vi "Get Biometry Data Path.vi"(8 "error in (no error)":errorcluster caption="错误输入（无错误）", 9 "Display Parameter":T1(ring), 10 "condition":string, 11 "connection reference":T2) -> (0 "error out":errorcluster caption="错误输出", 2 "Data Path Output":string[](array[string]))   [LabVIEW 2015, in "Utility VIs.lvlib"]
doc: "该模板用于创建子VI。"
uses:
  Utility VIs.lvlib
  <vilib>/addons/database/Connection.llb/Conn ObjectReference.ctl
  Database Processing/Database Processing.lvlib
  <vilib>/addons/database/NI_Database_API.lvlib
panel:
  # "Busy"
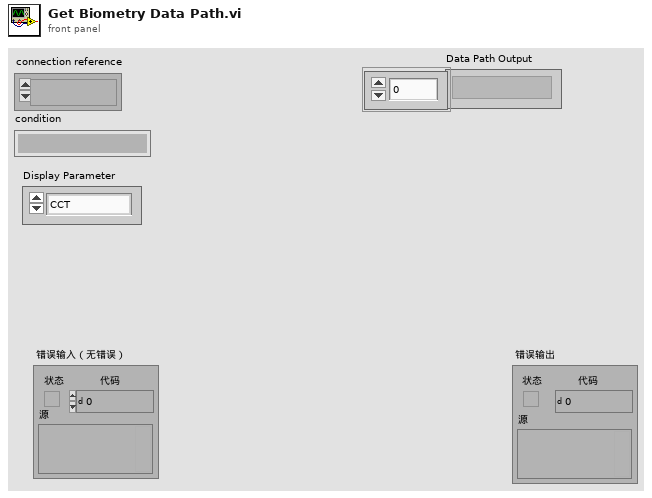
[diagram p1: front panel]
types:
  T1 = enum16{"CCT", "ACD", "LT", "RT", "AL", "PD", "WTW", "K_flat", "K_steep"}
  T2 = typedef "NI_Database_API.lvlib/Conn ObjectReference.ctl" = refnum<k1>
  T3 = typedef "Database Processing.lvlib/Biometry Attribute.ctl" = cluster{"Measure_ID":i64, "Measure_No":i64, "Ordinal":i64, "L_Or_R":string}
  T4 = typedef "Database Processing.lvlib/Biometry Data Path.ctl" = cluster{"Measure_ID":i64, "Ascan_data_Original":string, "picture_pupil_Original":string, "picture_WTW_Original":string, "Ascan_data_Processing":string, "picture_pupil_Processing":string, "picture_WTW_Processing":string, "picture_Processing_K":string, "picture_Processing_ALL":string}
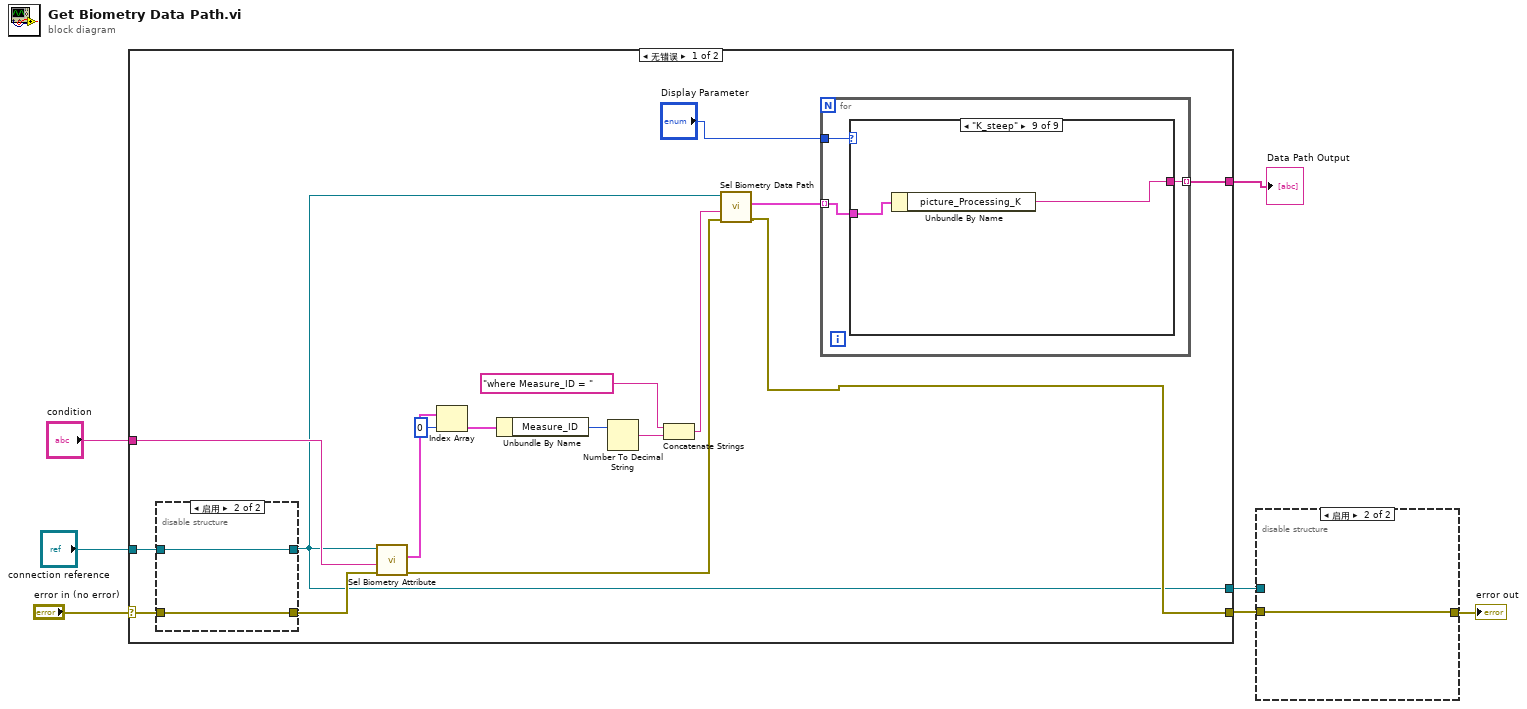
[diagram p0: block diagram]
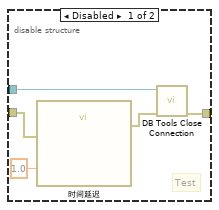
[diagram p2: hidden frame]
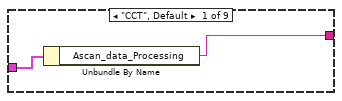
[diagram p3: hidden frame]
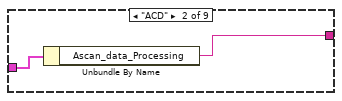
[diagram p4: hidden frame]
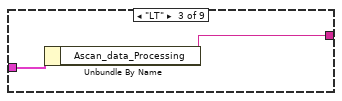
[diagram p5: hidden frame]
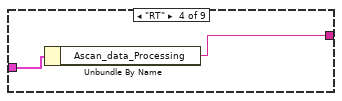
[diagram p6: hidden frame]
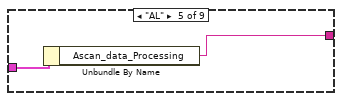
[diagram p7: hidden frame]
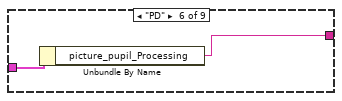
[diagram p8: hidden frame]
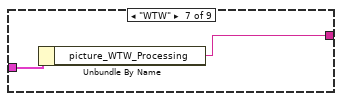
[diagram p9: hidden frame]
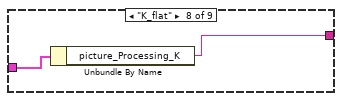
[diagram p10: hidden frame]
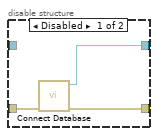
[diagram p11: hidden frame]
diagram:
  n1 = case shown="无错误" "error in (no error)" {
    selector: "error in (no error)" -> [w24 w52]
    tunnel: [w11 w52] -> w4
    tunnel: "connection reference" -> [w23 w51]
    tunnel: "condition" -> [w15 _]
    tunnel: [w10 w51] -> w2
    tunnel: [w9 _] -> w1
    frame No Error {
      n2 = disable-structure shown="启用" {
        disable-tunnel: w24 -> [w48 w49]
        disable-tunnel: w23 -> [_ w50]
        disable-tunnel: [w47 w50] -> w10
        disable-tunnel: [w46 w49] -> w17
        frame Disabled {
          n3 = call "Connect Database.vi"("error in (no error)"=w48) -> ("error out"=w46:errorcluster, "connection reference"=w47:T2)  [unwired: 9 in]
        }
        frame Enabled {
        }
      }
      n4 = call "Sel Biometry Attribute.vi"("error in (no error)"=w17, "condition"=w15, "connection reference"=w10) -> ("error out"=w12:errorcluster, "Biometry Attribute"=w16:T3[])  [unwired: 7 in]
      n5 = Index Array(array=w16, index=0 ("索引")) -> (element=w21:T3)
      n6 = Unbundle By Name(w21) -> ("Measure_ID"=w19:i64)
      n7 = Number To Decimal String(number=w19) -> (decimal integer string=w20:string)  [unwired: 1 in]
      n8 = Concatenate Strings("where Measure_ID = " ("字符串"), w20) -> (w13:string)
      n9 = call "Sel Biometry Data Path.vi"("error in (no error)"=w12, "condition"=w13, "connection reference"=w10) -> ("error out"=w11:errorcluster, "Biometry Data Path"=w8:T4[])  [unwired: 7 in]
      n10 = for {
        tunnel: "Display Parameter" -> [w27]
        tunnel: [w26] -> w9 mode=indexing
        tunnel: w8 -> [w25] mode=indexing
        n11 = case shown="\"K_steep\"" w27 {
          tunnel: w25 -> [w29 w31 w33 w35 w37 w39 w41 w43 w45]
          tunnel: [w28 w30 w32 w34 w36 w38 w40 w42 w44] -> w26
          frame "CCT", Default {
            n12 = Unbundle By Name(w29) -> ("Ascan_data_Processing"=w28:string)
          }
          frame "ACD" {
            n13 = Unbundle By Name(w31) -> ("Ascan_data_Processing"=w30:string)
          }
          frame "LT" {
            n14 = Unbundle By Name(w33) -> ("Ascan_data_Processing"=w32:string)
          }
          frame "RT" {
            n15 = Unbundle By Name(w35) -> ("Ascan_data_Processing"=w34:string)
          }
          frame "AL" {
            n16 = Unbundle By Name(w37) -> ("Ascan_data_Processing"=w36:string)
          }
          frame "PD" {
            n17 = Unbundle By Name(w39) -> ("picture_pupil_Processing"=w38:string)
          }
          frame "WTW" {
            n18 = Unbundle By Name(w41) -> ("picture_WTW_Processing"=w40:string)
          }
          frame "K_flat" {
            n19 = Unbundle By Name(w43) -> ("picture_Processing_K"=w42:string)
          }
          frame "K_steep" {
            n20 = Unbundle By Name(w45) -> ("picture_Processing_K"=w44:string)
          }
        }
      }
    }
    frame Error {
    }
  }
  "Data Path Output" <- w1
  n21 = disable-structure shown="启用" {
    disable-tunnel: w4 -> [w55 w58]
    disable-tunnel: [w57 w58] -> w3
    disable-tunnel: w2 -> [w56 _]
    frame Disabled {
      # "Test"
      n22 = call "时间延迟"("error in (no error)"=w55, "Delay Time (s)"=1.0) -> ("error out"=w54:errorcluster)  [unwired: 9 in]
      n23 = call <vilib>:"DB Tools Close Connection.vi"("error in (no error)"=w54, "connection reference"=w56) -> ("error out"=w57:errorcluster)  [unwired: 5 in]
    }
    frame Enabled {
    }
  }
  "error out" <- w3
